vi "write_params.vi"(8 "error in (no error)":errorcluster, 10 "params":T1={"n_clusters"=3.0, "svd_method"="randomized", "n_svd_vecs"={"n_svd_vecs_type"="None", "n_svd_int"=0.0}, "mini_batch"=FALSE, "init"={"init_type"="k-means++", "init_list"=[]}, "n_init"=10.0, "random_state"=0.0}, 11 "SpectralCoclustering in":refnum<class "SpectralCoclustering.lvclass">) -> (0 "error out":errorcluster, 3 "SpectralCoclustering out":refnum<class "SpectralCoclustering.lvclass">)   [LabVIEW 2020, in "SpectralCoclustering.lvclass"]
uses:
  SpectralCoclustering.lvclass
  Controls/spectral_coclustering_params.ctl
  SpectralCoclustering.lvclass/SpectralCoclustering.ctl
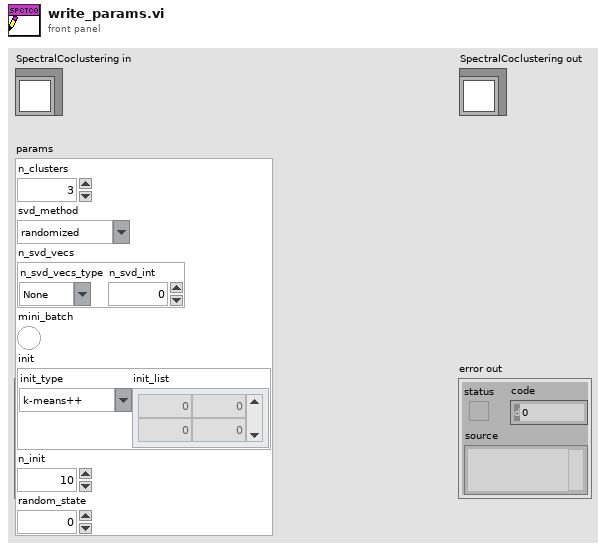
[diagram p1: front panel]
types:
  T1 = typedef "spectral_coclustering_params.ctl" = cluster{"n_clusters":dbl, "svd_method":string, "n_svd_vecs":cluster{"n_svd_vecs_type":string, "n_svd_int":dbl}, "mini_batch":bool, "init":cluster{"init_type":string, "init_list":dbl[][]}, "n_init":dbl, "random_state":dbl}
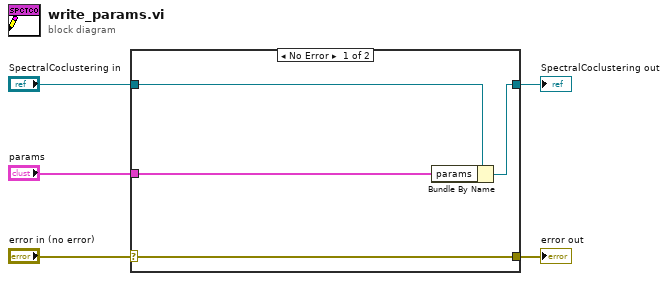
[diagram p0: block diagram]
diagram:
  n1 = case shown="No Error" "error in (no error)" {
    selector: "error in (no error)" -> [w9 w10]
    tunnel: [w9 w10] -> w4
    tunnel: [w7 w11] -> w2
    tunnel: "SpectralCoclustering in" -> [w8 w11]
    tunnel: "params" -> [w6 _]
    frame No Error {
      n2 = Bundle By Name(cluster=w8, "params"=w6) -> (w7:refnum<class "SpectralCoclustering.lvclass">)
    }
    frame Error {
    }
  }
  "error out" <- w4
  "SpectralCoclustering out" <- w2
